vi "Create Cal File Array (Dunk Tank).vi"(10 "Cal Log IN":string[][](array[string]), 11 "Available Channels":string[](array[string])) -> (1 "Cal Log OUT":string[][](array[string]))   [LabVIEW 2013]
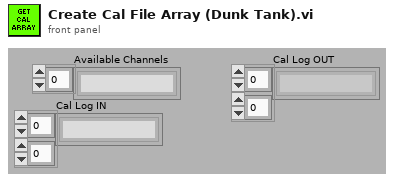
[diagram p1: front panel]
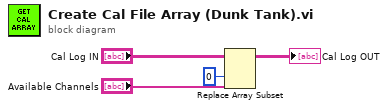
[diagram p0: block diagram]
diagram:
  n1 = Replace Array Subset(array="Cal Log IN", new element="Available Channels", index (col)=0 ("disabled index (col)")) -> (→"Cal Log OUT":string[][])  [unwired: 1 in]
